vi "AlliGator Update Menu.vi"(8 "Error In":errorcluster, 11 "Menu in":refnum<k9>) -> (0 "Error Out":errorcluster)   [LabVIEW 2021, in "AlliGator GUI.lvlib"]
doc: "Updates AlliGator menu upon activation, in order to set checkmarks and include dynamic menu items such as Python plugins."
uses:
  AlliGator GUI.lvlib
  AlliGator Globals.vi
  AlliGator Globals, Variables & Constants.lvlib
  AlliGator Python Plugins.lvlib
panel:
  # "see the AlliGator License on the block diagram (Ctrl+E or Window:Show Block Diagram)"
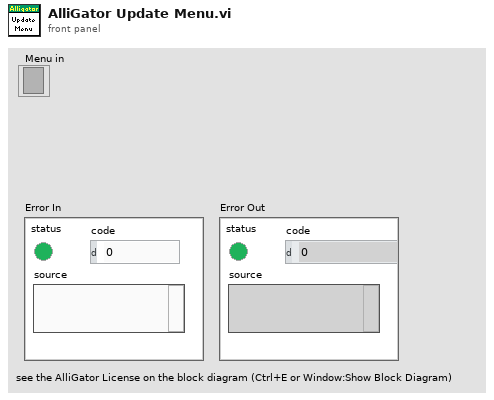
[diagram p1: front panel]
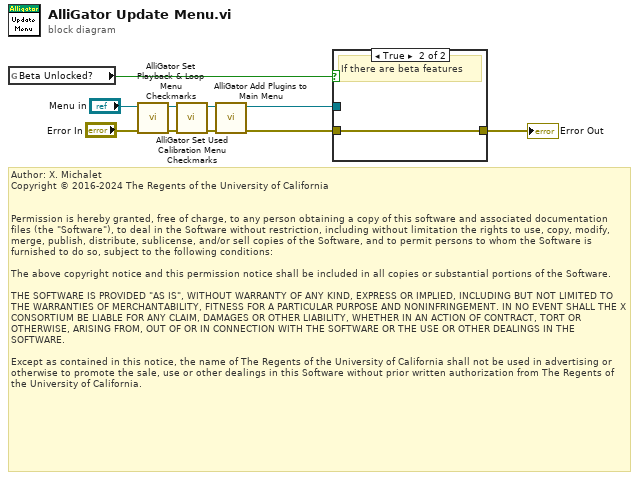
[diagram p0: block diagram]
diagram:
  # "Author: X. Michalet\nCopyright © 2016-2024 The Regents of the University of California\n \n\nPermission is hereby granted, free of charge, to any person obtaining a copy of this software and associated documentation files (the \"Software\"), to deal in the Software without restriction, including without limitation the rights to use, copy, modify, merge, publish, distribute, sublicense, and/or sell copies of the Software, and to permit persons to whom the Software is furnished to do so, subject to the following conditions:\n\nThe above copyright notice and this permission notice shall be included in all copies or substantial portions of the Software.\n\nTHE SOFTWARE IS PROVIDED \"AS IS\", WITHOUT WARRANTY OF ANY KIND, EXPRESS OR IMPLIED, INCLUDING BUT NOT LIMITED TO THE WARRANTIES OF MERCHANTABILITY, FITNESS FOR A PARTICULAR PURPOSE AND NONINFRINGEMENT. IN NO EVENT SHALL THE X CONSORTIUM BE LIABLE FOR ANY CLAIM, DAMAGES OR OTHER LIABILITY, WHETHER IN AN ACTION OF CONTRACT, TORT OR OTHERWISE, ARISING FROM, OUT OF OR IN CONNECTION WITH THE SOFTWARE OR THE USE OR OTHER DEALINGS IN THE SOFTWARE.\n\nExcept as contained in this notice, the name of The Regents of the University of California shall not be used in advertising or otherwise to promote the sale, use or other dealings in this Software without prior written authorization from The Regents of the University of California."
  n1 = global read "AlliGator Globals.vi" "Beta Unlocked?"() -> (w8:bool)
  n2 = call "AlliGator Set Playback & Loop Menu Checkmarks.vi"("Error In"="Error In", "Menu in"="Menu in") -> ("Error Out"=w3:errorcluster, "Menu out"=w4:refnum<k9>)  [unwired: 8 in]
  n3 = call "AlliGator Set Used Calibration Menu Checkmarks.vi"("Error In"=w3, "Menu in"=w4) -> ("Error Out"=w2:errorcluster, "Menu out"=w1:refnum<k9>)  [unwired: 8 in]
  n4 = call "AlliGator Add Plugins to Main Menu.vi"("error in (no error)"=w2, "Menu in"=w1) -> ("error out"=w7:errorcluster, "Menu out"=w5:refnum<k9>)  [unwired: 8 in]
  n5 = case shown="True" w8 {
    tunnel: w7 -> [w11 w12]
    tunnel: [w11 w12] -> w6
    tunnel: w5 -> [_ _]
    frame False {
    }
    frame True {
      # "If there are beta features"
    }
  }
  "Error Out" <- w6
